vi "PipBoy_SetIconName.vi"(6 "DrawIcon?":bool, 8 "error in (no error)":errorcluster, 9 "Icon to draw":i32, 10 "Function":string, 11 "VisaPic32In":refnum<visa-resource-name>) -> (0 "error out":errorcluster, 3 "VisaPic32Out":refnum<visa-resource-name>)   [LabVIEW 2014]
uses:
  <vilib>/Utility/error.llb/Error Cluster From Error Code.vi
  <vilib>/ErrorRing/Error Ring.xnode
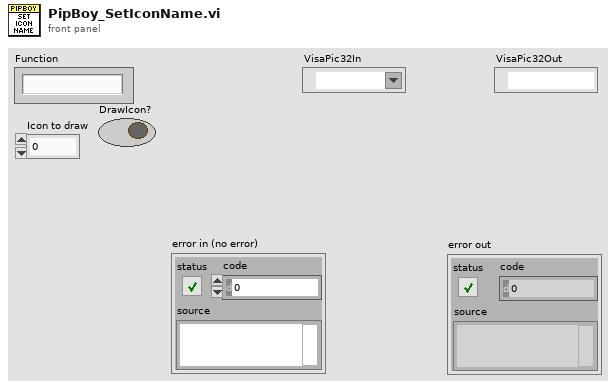
[diagram p1: front panel]
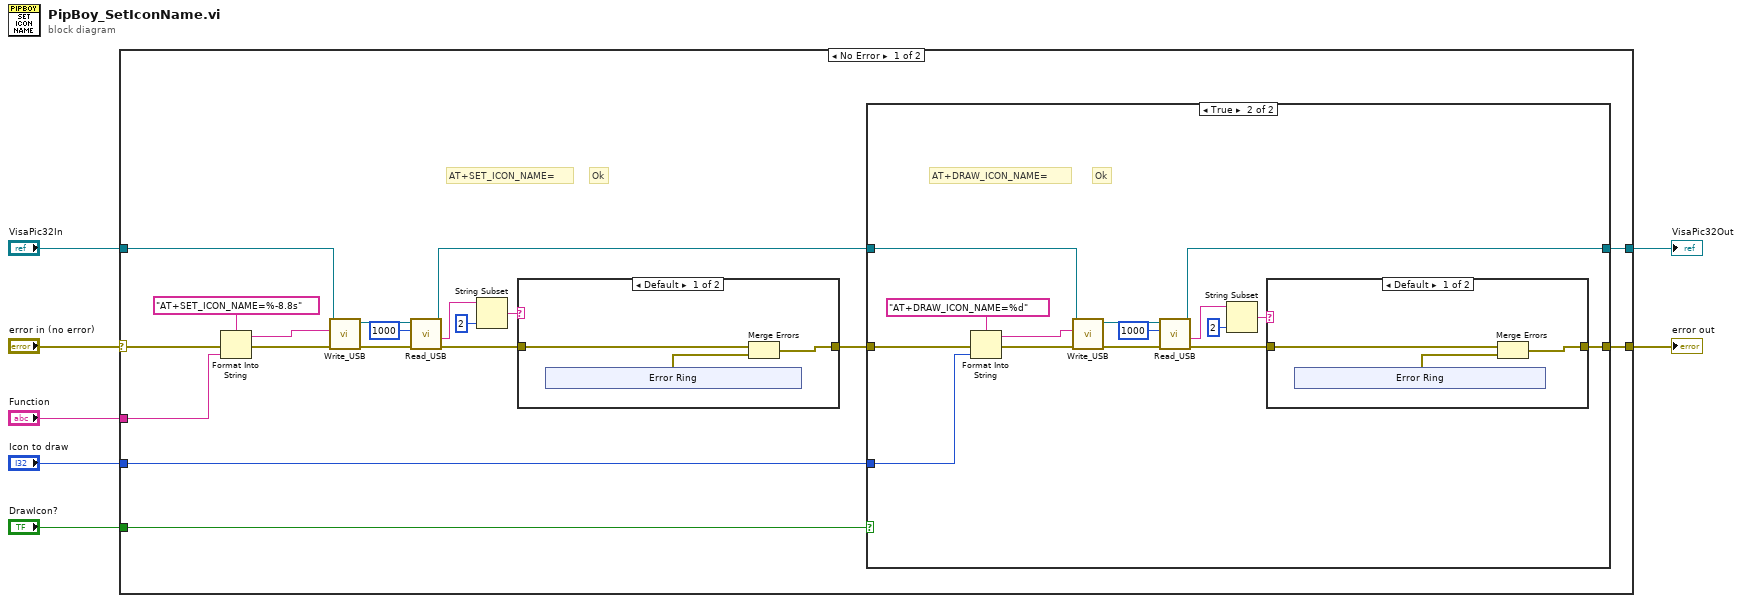
[diagram p0: block diagram]
diagram:
  n1 = case shown="No Error" "error in (no error)" {
    selector: "error in (no error)" -> [w21 w63]
    tunnel: [w13 w63] -> w6
    tunnel: [w15 w62] -> w5
    tunnel: "VisaPic32In" -> [w23 w62]
    tunnel: "Function" -> [w8 _]
    tunnel: "Icon to draw" -> [w14 _]
    tunnel: "DrawIcon?" -> [w9 _]
    frame No Error {
      # "Ok"
      # "AT+SET_ICON_NAME="
      n2 = Format Into String(format string="AT+SET_ICON_NAME=%-8.8s" ("buffer d'écriture"), error in=w21, w8) -> (resulting string=w18:string, error out=w20:errorcluster)  [unwired: 1 in]
      n3 = call "Write_USB.vi"("entrée d'erreur"=w20, "buffer d'écriture"=w18, "Nom de ressource VISA"=w23) -> ("sortie d'erreur"=w24:errorcluster, "Nom de ressource VISA en sortie"=w25:refnum<visa-resource-name>)  [unwired: 7 in]
      n4 = call "Read_USB.vi"("entrée d'erreur"=w24, "timeout (0)"=u32 1000, "Nom de ressource VISA"=w25) -> ("sortie d'erreur"=w22:errorcluster, "chaîne en sortie"=w10:string, "Nom de ressource VISA en sortie"=w16:refnum<visa-resource-name>)  [unwired: 6 in]
      n5 = String Subset(string=w10, length (rest)=2 ("length (rest)")) -> (substring=w11:string)  [unwired: 1 in]
      n6 = case shown="Default" w11 {
        tunnel: [w54 w61] -> w17
        tunnel: w22 -> [w55 w61]
        frame Default {
          n7 = xnode "Error Ring"() -> ("error out"=w53:errorcluster)
          n8 = Merge Errors(w55, w53) -> (w54:errorcluster)
        }
        frame "OK" {
        }
      }
      n9 = case shown="True" w9 {
        tunnel: w17 -> [w28 w40]
        tunnel: w16 -> [w27 w37]
        tunnel: [w27 w36] -> w15
        tunnel: w14 -> [_ w34]
        tunnel: [w28 w32] -> w13
        frame False {
        }
        frame True {
          # "Ok"
          # "AT+DRAW_ICON_NAME="
          n10 = Format Into String(format string="AT+DRAW_ICON_NAME=%d", error in=w40, w34) -> (resulting string=w35:string, error out=w39:errorcluster)  [unwired: 1 in]
          n11 = call "Write_USB.vi"("entrée d'erreur"=w39, "buffer d'écriture"=w35, "Nom de ressource VISA"=w37) -> ("sortie d'erreur"=w43:errorcluster, "Nom de ressource VISA en sortie"=w42:refnum<visa-resource-name>)  [unwired: 7 in]
          n12 = call "Read_USB.vi"("entrée d'erreur"=w43, "timeout (0)"=u32 1000, "Nom de ressource VISA"=w42) -> ("sortie d'erreur"=w33:errorcluster, "chaîne en sortie"=w30:string, "Nom de ressource VISA en sortie"=w36:refnum<visa-resource-name>)  [unwired: 6 in]
          n13 = String Subset(string=w30, length (rest)=2 ("length (rest)")) -> (substring=w29:string)  [unwired: 1 in]
          n14 = case shown="Default" w29 {
            tunnel: [w45 w52] -> w32
            tunnel: w33 -> [w46 w52]
            frame Default {
              n15 = xnode "Error Ring"() -> ("error out"=w44:errorcluster)
              n16 = Merge Errors(w46, w44) -> (w45:errorcluster)
            }
            frame "OK" {
            }
          }
        }
      }
    }
    frame Error {
    }
  }
  "error out" <- w6
  "VisaPic32Out" <- w5
